vi "binary record both ch_v01_loop.vi"(4 "Record":bool, 8 "reference":refnum<vi>, 9 "path":path, 10 "wfm":i16[][](array[numeric]), 11 "Chan 1 params":T1) -> ()   [LabVIEW 2013]
panel:
  out "error out":errorcluster
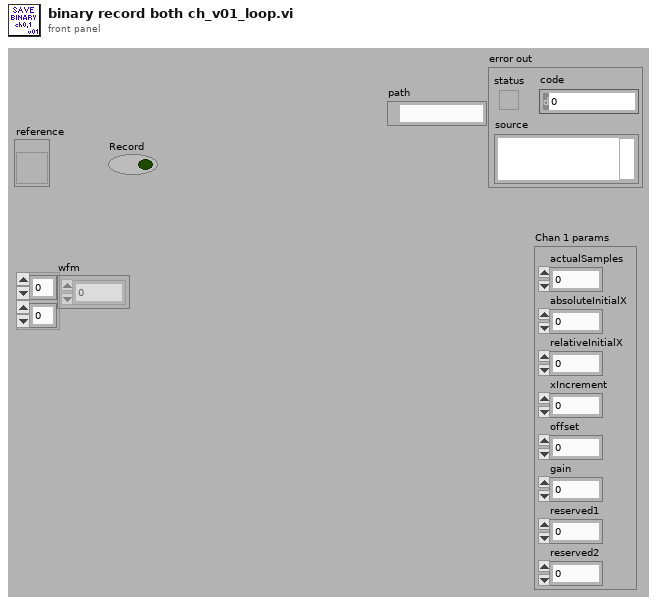
[diagram p1: front panel]
types:
  T1 = cluster{"actualSamples":i32, "absoluteInitialX":dbl, "relativeInitialX":dbl, "xIncrement":dbl, "offset":dbl, "gain":dbl, "reserved1":dbl, "reserved2":dbl}
  T2 = enum16{"open", "replace", "create", "open or create", "replace or create", "replace or create with confirmation"}
  T3 = enum16{"big-endian, network order", "native, host order", "little-endian"}
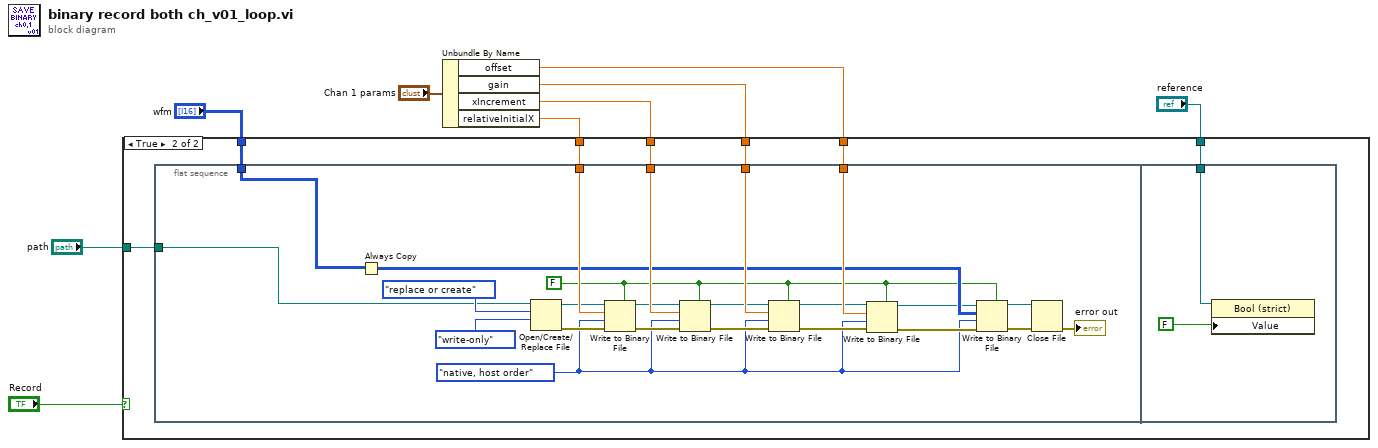
[diagram p0: block diagram]
diagram:
  n1 = Unbundle By Name("Chan 1 params") -> ("offset"=w2:dbl, "gain"=w3:dbl, "xIncrement"=w4:dbl, "relativeInitialX"=w5:dbl)
  n2 = case shown="True" "Record" {
    tunnel: "wfm" -> [_ w16]
    tunnel: w5 -> [_ w15]
    tunnel: w4 -> [_ w14]
    tunnel: w3 -> [_ w13]
    tunnel: w2 -> [_ w12]
    tunnel: "reference" -> [_ w11]
    tunnel: "path" -> [_ w10]
    frame False {
    }
    frame True {
      n3 = flat-sequence {
        tunnel: w16 -> [w19]
        tunnel: w15 -> [w40]
        tunnel: w14 -> [w39]
        tunnel: w13 -> [w38]
        tunnel: w12 -> [w37]
        tunnel: w10 -> [w17]
        tunnel: w11 -> [w41]
        frame #0 {
          w20 = FALSE ("prepend array or string size? (T)")
          w21 = T3."native, host order" ("byte order (0:big-endian, network order)")
          n4 = Always Copy(1:w19) -> (0:w34:i16[][])
          n5 = Open/Create/Replace File(file path (use dialog)=w17, operation (0:open)=T2."replace or create", access (0:read/write)=enum16{"read/write", "read-only", "write-only"}."write-only") -> (refnum out=w33:refnum<file>, error out=w32:errorcluster)  [unwired: 1 in, 3 out]
          n6 = Write to Binary File(file (use dialog)=w33, data=w40, error in=w32, 5:w20, 9:w21) -> (refnum out=w31:refnum<file>, error out=w30:errorcluster)  [unwired: 2 out]
          n7 = Write to Binary File(file (use dialog)=w31, data=w39, error in=w30, 5:w20, 9:w21) -> (refnum out=w29:refnum<file>, error out=w25:errorcluster)  [unwired: 2 out]
          n8 = Write to Binary File(file (use dialog)=w29, data=w38, error in=w25, 5:w20, 9:w21) -> (refnum out=w28:refnum<file>, error out=w24:errorcluster)  [unwired: 2 out]
          n9 = Write to Binary File(file (use dialog)=w28, data=w37, error in=w24, 5:w20, 9:w21) -> (refnum out=w27:refnum<file>, error out=w23:errorcluster)  [unwired: 2 out]
          n10 = Write to Binary File(file (use dialog)=w27, data=w34, error in=w23, 5:w20, 9:w21) -> (refnum out=w26:refnum<file>, error out=w22:errorcluster)  [unwired: 2 out]
          n11 = Close File(refnum=w26, error in=w22) -> (error out=→"error out":errorcluster)  [unwired: 1 out]
        }
        frame #1 {
          n12 = property on="Property Node" class="Bool (strict)"(reference=w41, "Value"=FALSE ("Boolean")) -> ()  [unwired: 1 in, 2 out]
        }
      }
    }
  }
